vi "Misura res.vi"(6 "Scala per ramo":i32[](array[numeric]), 8 "String":string="Misura resistenze.. ", 9 "Status":refnum<vi>, 11 "N°rami":i32=3) -> (1 "temperature amb":dbl[](array[numeric]), 2 "Valori res (ohm)":dbl[](array[numeric]), 3 "Rmedia (ohm)":dbl format="%0.2f")   [LabVIEW 2019]
uses:
  cDAQ_PLC Folder/cDAQ/SET ARRAY DO.ctl
  cDAQ_PLC Folder/cDAQ/SET SINGLE DO.ctl
  cDAQ_PLC Folder/cDAQ/DO List.ctl
  <vilib>/Analysis/baseanly.llb/Mean (DBL).vi
  Global_All_Data.vi
  Global_scelta_linea.vi
  Resistomat/Stop lettura res.vi
  Global prova in corso.vi
  <vilib>/Analysis/NI_AALBase.lvlib
panel:
  in  "Scala di misura":u16
  out "Message":string
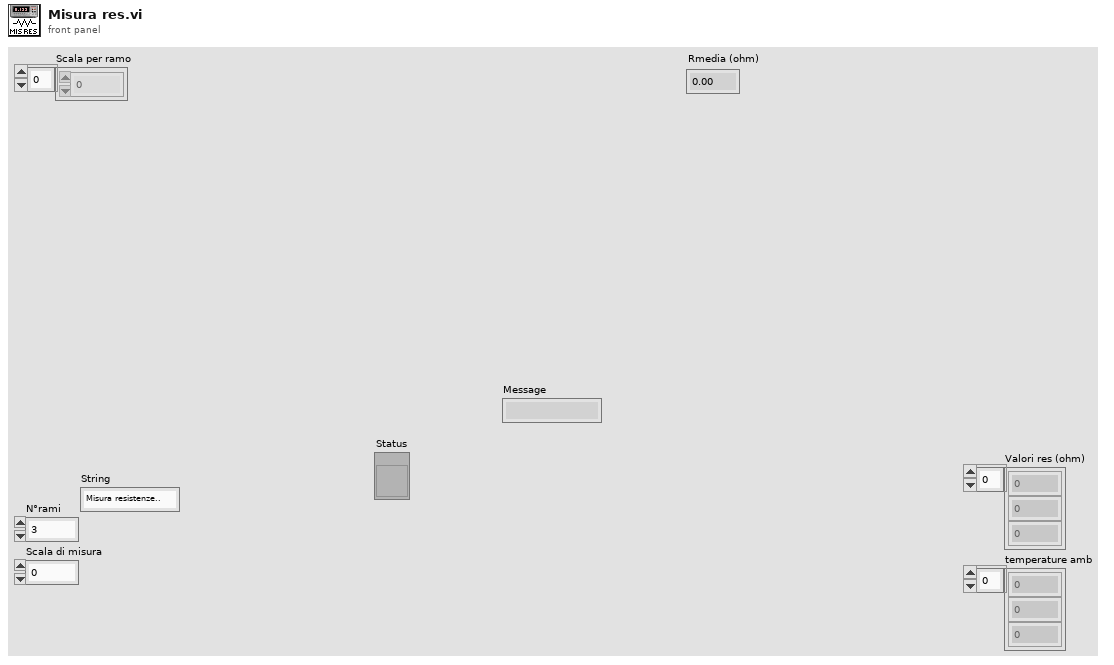
[diagram p1: front panel]
types:
  T1 = typedef "SET ARRAY DO.ctl" = T2[]
  T2 = typedef "SET SINGLE DO.ctl" = cluster{"DO":T3, "Value":bool}
  T3 = typedef "DO List.ctl" = enum16{"OFF: ALL DO", "*ABILITA freno 1", "*ABILITA freno 2", "*ABILITA freno 3", "*START freno 1", "*START freno 2", "*START freno 3", "*STOP freno 1", "*STOP freno 3", "*STOP freno 2", "*Senso rot freno 1", "*Senso rot freno 2", "*Senso rot freno 3", "*Ctrl velocità freno 1", "*Ctrl velocità freno 2", "*Ctrl velocità freno 3", "*Ctrl coppia freno 1", "*Ctrl coppia freno 2", "*Ctrl coppia freno 3", "*ABILITA alimentatore 1", "*ABILITA alimentatore 2", "*ABILITA alimentatore 3", "*ABILITA alimentatore 4", "*START alimentatore 1", "*START alimentatore 2", "*START alimentatore 3", "*START alimentatore 4", "*STOP alimentatore 1", "*STOP alimentatore 2", "*STOP alimentatore 3", "*STOP alimentatore 4", "SENSO ROT alimentatore 1", "SENSO ROT alimentatore 2", "Abilita LEM 1000A", "Abilita LEM 300A", "Abilita sensori EXT WT", "B1 Seleziona linea 1", "B1 Seleziona linea 2", "B1 Seleziona linea 3", "B1 Seleziona linea 4", "B1 Seleziona linea 5", "B2 Seleziona linea 1", "B2 Seleziona linea 2", "B2 Seleziona linea 3", "B2 Seleziona linea 4", "B2 Seleziona linea 5", "*Reset allarmi", "*Start potenza AC", "*Stop potenza AC", "*Start potenza DC", "*Stop potenza DC", "*Start potenza DC eccit", "*Stop pontenza DC eccit", "Bypass res meter", "2nd canale res meter", "Enable res meter", "*Abilit teler ramo WT", "*Abil teler ramo princ Resit", "*Abil teler ramo 1 Resist", "*Abil teler ramo 2 Resist", "*Abil teler ramo 3 Resist", "*Abil cortocirc avvolgim", "*Controllo torsiometro B1", "*Controllo Torsiom B2", "*Scala torsiometro B1", "*Scala torsiometro B2", "*Collaudo in corso", "*Allarme presente", "Abilitazione elettroserratura", "Exit", "*Abilita collaudo", "*Abilita potenza trifase", "*Abilita potenza monofase", "*Abilita potenza DC", "*Abilita potenza DC eccit", "*Disabilita teleruttori potenza", "Set teleruttori prova a freddo", "Prova a freddo monofase", "Watchdog", "Forza DO PLC 3", "Forza DO PLC 2", "Forza DO PLC 1", "Forza DO cDAQ", "Scala 2000(T) 200(F) res meter", "Seleziona banco 1", "Seleziona banco 2", "Comando azionam in blocco", "Comando azionam reset", "Sensibilità freno 16 32 nm", "Reset Allarmi", "Carico res - Ramo 1", "Carico res - Ramo 2", "Carico res - Ramo 3", "Carico res - Ramo 4", "Carico res - Ramo 5", "Carico res - Ramo 6", "Carico res - Ramo 7", "Carico res - Ramo 8", "Carico res - Ramo 9", "Carico res - Ramo 10", "Carico res - Ramo 11", "Carico res - Start ventilatore", "Carico res - Stop ventilatore", "Abilita potenza solo freno", "Abilita AFE + freno trasc", "Abilita potenza carico resistivo", "Chiudi potenza AFE", "Apri potenza AFE", "Start AFE", "Config Banco2 TDE", "Misura diretto WT", "Ripristina centralina protezioni", "Abilita Scrittura Dati Keb"}
  T4 = cluster{"Array of elements":cluster{"String":string, "variant":variant}[], "Single element":cluster{"String":string, "variant":variant}, "enque at\nopposite end (F)":bool, "no replications (F)":bool}
  T5 = typedef "Cluster MISURE.ctl" = cluster{"MISURE NM":T6, "MISURE ALL":T7}
  T6 = typedef "MISURE NM.ctl" = cluster{"Banco":string, "Anno":string, "Numero":string, "Ntabella":string, "Misura":string, "Tipo Prova":string, "ProgressivoAcq":string, "Descrizione":string, "Data_ora":string, "t. acq [h:m:s]":string, "t. acq [min]":string, "t. acq [s]":string, "n [rpm]":string, "f [Hz]":string, "U1[V]":string, "U2 [V]":string, "U3 [V]":string, "U123_media [V]":string, "I1[A]":string, "I2[A]":string, "I3[A]":string, "I123_media [A]*I":string, "I_123_sbil [%]":string, "Ulin[V]":string, "Uc [V]":string, "Uaux [V]":string, "Ilin[A]*I":string, "Imar[A]":string, "Iaux[A]":string, "Uarm[V]":string, "Uecc[V]":string, "Iarm[A]*I":string, "Iecc[A]":string, "pf":string, "P1 [W]":string, "P1 [kW]":string, "Q [VAR]":string, "Q [kVAR]":string, "S [VA]":string, "S [kVA]":string, "P1arm[W]":string, "P1ecc[W]":string, "Parm[kW]":string, "P1ecc[kW]":string, "Cond[uF]":string, "P1_linea_6fili[W]":string, "P1_linea_6fili[kW]":string, "eta_gr_6fili [%]":string, "eta_inverter_6fili [%]":string, "pf_linea_6fili":string, "U4 [V]":string, "U5 [V]":string, "U6 [V]":string, "U456_media [V]":string, "I4 [A]":string, "I5 [A]":string, "I6 [A]":string, "I456_media [A]":string, "C [Nm]*C":string, "Cric [Nm]":string, "Cric\\Cnom":string, "Iric[A]":string, "Iric\\Inom":string, "P2_mecc [W]":string, "P2_mecc [kW]":string, "eta motore [%]":string, "Scorr[%]":string, "Tamb[°C]":string, "R1[ohm]":string, "R2[ohm]":string, "R3[ohm]":string, "Rmedia[ohm]":string, "DT_R1[°C]":string, "DT_R2[°C]":string, "DT_R3[°C]":string, "DT_media[°C]":string, "R_marcia[ohm]":string, "R_aux[ohm]":string, "DT_marcia[°C]":string, "DT_aux[°C]":string, "R_Arm[ohm]":string, "R_Ecc[ohm]":string, "DT_Arm[°C]":string, "DT_Ecc[°C]":string, "TambFreddo[°C]":string, "R1_freddo[ohm]":string, "R2_freddo[ohm]":string, "R3_freddo[ohm]":string, "Rmedia_freddo[ohm]":string, "R_Marcia_freddo[ohm]":string, "R_Aux_freddo[ohm]":string, "R_Arm_freddo[ohm]":string, "R_Ecc_freddo[ohm]":string, "TC1 [°C]":string, "TC2 [°C]":string, "TC3 [°C]":string, "TC4 [°C]":string, "TC5 [°C]":string, "TC6 [°C]":string, "TC7 [°C]":string, "TC8 [°C]":string, "PT1000_1[°C]":string, "PT1000_2[°C]":string, "PT1000_3[°C]":string, "Vdc eccitatrice[V]":string, "Idc eccitatrice[A]":string, "Vdc rotore[V]":string, "Idc rotore[A]":string, "Vac rotore[V]":string, "Iac rotore[V]":string, "V dinamo[V]":string, "Portata Q":string, "Pressione H":string, "U1'[V]":string, "U2'[V]":string, "U3'[V]":string, "I1'[A]":string, "I2'[A]":string, "I3'[A]":string, "U''R-N":string, "U''S-N":string, "U'' T-N":string, "U''R-S":string, "U''R-T":string, "U''S-T":string, "I1''[A]":string, "I2''[A]":string, "I3''[A]":string, "F''[Hz]":string, "P''[kW]":string, "CosFi''":string, "PT1000_4[°C]":string, "Scorta 3":string}
  T7 = typedef "Cluster misure ALL.ctl" = cluster{"Cluster READ NI":T8, "MISURE WT":T11, "Resistenze Resistomat":T12, "INTERFACCIA":T13, "FREDDO resistomat":cluster{"Res Ch1":dbl, "Res Ch2":dbl, "tAMB":dbl, "Res Ch3":dbl}, "STATO PLC 1":T18, "Res Ch2":dbl, "Res Ch2 2":dbl, "FREDDO res meter":cluster{"Res Ch1":dbl, "Res Ch2":dbl, "tAMB":dbl, "Res Ch3":dbl}, "Resistenze Res Meter":T12, "READ SINUS PENTA":T22, "STATO PLC 2":T23, "STATO PLC 3":T27, "DCREG":T31}
  T8 = typedef "Cluster NI.ctl" = cluster{"AI (0-10V)":cluster{"AI 0":dbl, "AI 1":dbl, "AI 2":dbl, "AI 3":dbl, "AI 4":dbl, "AI 5":dbl, "AI 6":dbl, "AI 7":dbl, "AI 8":dbl, "AI 9":dbl, "AI 10":dbl, "AI 11":dbl, "AI 12":dbl, "AI 13":dbl, "AI 14":dbl, "AI 15":dbl, "AI 16":dbl, "AI 17":dbl, "AI 18":dbl, "AI 19":dbl, "AI 20":dbl, "AI 21":dbl, "AI 22":dbl, "AI 23":dbl, "AI 24":dbl, "AI 25":dbl, "AI 26":dbl, "AI 27":dbl, "AI 28":dbl, "AI 29":dbl, "AI 30":dbl, "AI 31":dbl}, "StatoAO_Cdaq[0-10V]":cluster{"AO 1":dbl, "AO 2":dbl, "AO 3":dbl, "AO 4":dbl}, "Contatori [rpm]":cluster{"RPM 1":dbl, "RPM 2":dbl}, "StatoAO_Cdaq [4-20mA]":T9, "StatoDO_Cdaq":T10, "DI":cluster{"Scorta 0":bool, "Scorta 1":bool, "Scorta 2":bool, "Scorta 3":bool, "Scorta 4":bool, "Scorta 5":bool, "Scorta 6":bool, "Scorta 7":bool, "Scorta 8":bool, "Scorta 9":bool, "Scorta 10":bool, "Scorta 11":bool, "Scorta 12":bool, "Scorta 13":bool, "Scorta 14":bool, "Scorta 15":bool, "Scorta 16":bool, "Scorta 17":bool, "Scorta 18":bool, "Scorta 19":bool, "Scorta 20":bool, "Scorta 21":bool, "Scorta 22":bool, "Scorta 23":bool, "Scorta 24":bool, "Scorta 25":bool, "Scorta 26":bool, "Scorta 27":bool, "Scorta 28":bool, "Scorta 29":bool, "Scorta 30":bool, "Scorta 31":bool}, "AI (4-20mA)":cluster{"AI 0":dbl, "AI 1":dbl, "AI 2":dbl, "AI 3":dbl, "AI 4":dbl, "AI 5":dbl, "AI 6":dbl, "AI 7":dbl, "AI 8":dbl, "AI 9":dbl, "AI 10":dbl, "AI 11":dbl, "AI 12":dbl, "AI 13":dbl, "AI 14":dbl, "AI 15":dbl}, "TC [°C]":cluster{"tc 1":dbl, "tc 2":dbl, "tc 3":dbl, "tc 4":dbl}}
  T9 = typedef "StatoAO_cdaq.ctl" = cluster{"Cdaq_AO [0-10V] 0":dbl, "Cdaq_AO [0-10V] 1":dbl, "Cdaq_AO [0-10V] 2":dbl, "Cdaq_AO [0-10V] 3":dbl, "Cdaq_AO [4-20mA] 0":dbl, "Cdaq_AO [4-20mA] 1":dbl, "Cdaq_AO [4-20mA] 2":dbl, "Cdaq_AO [4-20mA] 3":dbl, "Cdaq_AO [4-20mA] 4":dbl, "Cdaq_AO [4-20mA] 5":dbl, "Cdaq_AO [4-20mA] 6":dbl, "Cdaq_AO [4-20mA] 7":dbl}
  T10 = typedef "statoDO_Cdaq.ctl" = cluster{"Scorta 0":bool, "Scorta 1":bool, "Scorta 2":bool, "Scorta 3":bool, "Scorta 4":bool, "Scorta 5":bool, "Scorta 6":bool, "Scorta 7":bool, "Scorta 8":bool, "Scorta 9":bool, "Scorta 10":bool, "Scorta 11":bool, "Scorta 12":bool, "Scorta 13":bool, "Scorta 14":bool, "Scorta 15":bool, "Scorta 16":bool, "Scorta 17":bool, "Scorta 18":bool, "Scorta 19":bool, "Scorta 20":bool, "Scorta 21":bool, "Scorta 22":bool, "Scorta 23":bool, "Scorta 24":bool, "Scorta 25":bool, "Scorta 26":bool, "Scorta 27":bool, "Scorta 28":bool, "Scorta 29":bool, "Scorta 30":bool, "Scorta 31":bool}
  T11 = typedef "MISURE WT.ctl" = cluster{"URMS 1":dbl, "IRMS 1":dbl, "P 1":dbl, "S 1":dbl, "Q 1":dbl, "LAMBDA 1":dbl, "PHI 1":dbl, "F U 1":dbl, "F I 1":dbl, "NONE 1":dbl, "URMS 2":dbl, "IRMS 2":dbl, "P 2":dbl, "S 2":dbl, "Q 2":dbl, "LAMBDA 2":dbl, "PHI 2":dbl, "F U 2":dbl, "F I 2":dbl, "NONE 2":dbl, "URMS 3":dbl, "IRMS 3":dbl, "P 3":dbl, "S 3":dbl, "Q 3":dbl, "LAMBDA 3":dbl, "PHI 3":dbl, "F U 3":dbl, "F I 3":dbl, "NONE 3":dbl, "URMS 4":dbl, "IRMS 4":dbl, "P 4":dbl, "S 4":dbl, "Q 4":dbl, "LAMBDA 4":dbl, "PHI 4":dbl, "F U 4":dbl, "F I 4":dbl, "NONE 4":dbl, "URMS 5":dbl, "IRMS 5":dbl, "P 5":dbl, "S 5":dbl, "Q 5":dbl, "LAMBDA 5":dbl, "PHI 5":dbl, "F U 5":dbl, "F I 5":dbl, "NONE 5":dbl, "URMS 6":dbl, "IRMS 6":dbl, "P 6":dbl, "S 6":dbl, "Q 6":dbl, "LAMBDA 6":dbl, "PHI 6":dbl, "F U 6":dbl, "F I 6":dbl, "NONE 6":dbl, "URMS SIGMA":dbl, "IRMS SIGMA":dbl, "P SIGMA":dbl, "S SIGMA":dbl, "Q SIGMA":dbl, "LAMBDA SIGMA":dbl, "PHI SIGMA":dbl, "F U SIGMA":dbl, "F I SIGMA":dbl, "NONE 7":dbl, "URMS SIGMB":dbl, "IRMS SIGMB":dbl, "P SIGMB":dbl, "S SIGMB":dbl, "Q SIGMB":dbl, "LAMBDA SIGMB":dbl, "PHI SIGMB":dbl, "F U SIGMB":dbl, "F I SIGMB":dbl, "NONE 8":dbl, "URMS SIGMC":dbl, "IRMS SIGMC":dbl, "P SIGMC":dbl, "S SIGMC":dbl, "Q SIGMC":dbl, "LAMBDA SIGMC":dbl, "PHI SIGMC":dbl, "F U SIGMC":dbl, "F I SIGMC":dbl, "NONE 9":dbl, "SPEED":dbl, "TORQUE[Nm]":dbl, "Pmecc[kW]":dbl}
  T12 = typedef "ClusterRes.ctl" = cluster{"Res Ch1":dbl, "Res Ch2":dbl, "Res Ch3":dbl, "Tamb":dbl}
  T13 = typedef "INTERFACCIA.ctl" = cluster{"AI":cluster{"Portate":T14[], "Pressioni":T14[], "Coppie[Nm]":T14[], "Valvole prop %":T14[], "RPM":T14[], "Livelli":T14[], "Temperature":T14[], "Riferimenti %":T14[], "TENSIONI":T14[], "CORRENTI":T14[]}, "DI (logici)":cluster{"Start da pulsantiera":bool, "Stop da pulsantiera":bool, "Reset da pulsantiera":bool, "Sistema OK":bool, "Collaudo abilitato":bool, "Potenza trifase abilitata":bool, "Potenza monofase abilitata":bool, "Potenza DC abilitata":bool, "Potenza DC ECC abilitata":bool, "Start alimentazione AC":bool, "Start alimentazione DC":bool, "Start DC eccitazione":bool, "Teleruttore WT abilitato":bool, "Teleruttore Resistomat abilitato":bool, "Teleruttore corto fasi":bool, "Ramo 1 resistomat":bool, "Ramo 2 resistomat":bool, "Ramo 3 resistomat":bool, "B1 Scelta linea elettrica 1":bool, "B1 Scelta linea elettrica 2":bool, "B1 Scelta linea elettrica 3":bool, "B1 Scelta linea elettrica 4":bool, "B1 Scelta linea elettrica 5":bool, "B2 Scelta linea elettrica 1":bool, "B2 Scelta linea elettrica 2":bool, "B2 Scelta linea elettrica 3":bool, "B2 Scelta linea elettrica 4":bool, "B2 Scelta linea elettrica 5":bool, "Rotore bloccato 1":bool, "Rotore bloccato 2":bool, "FRENO 1 abilitato":bool, "FRENO 1 run":bool, "FRENO 1 senso rotaz":bool, "FRENO 1 ctrl velocità":bool, "FRENO 2 abilitato":bool, "FRENO 2 run":bool, "FRENO 2 senso rotaz":bool, "FRENO 2 ctrl velocità":bool, "ALIM 1 abilitato":bool, "ALIM 1 run":bool, "ALIM 2 abilitato":bool, "ALIM 2 run":bool, "ALIM 3 abilitato":bool, "ALIM 3 run":bool, "FRENO 1 ctrl coppia":bool, "FRENO 2 ctrl coppia":bool, "FRENO 3 ctrl coppia":bool, "DI (logici) aggiuntivi impianto":cluster{"Solo freno abilitato":bool, "Carico resistivo abilitato":bool, "AFE+freno abilitato":bool, "Protezioni chiuse":bool, "Start potenza AFE":bool, "AFE in marcia":bool}, "Misura corrente diretta WT":bool, "Misura corrente sens ext":bool, "Sens ext abilitati":bool}, "AO non scalati":T16, "AO scalati":T16, "DO (logici)":T17}
  T14 = typedef "ClusterMisura_e_Unità_INPUT.ctl" = cluster{"Misura":dbl, "UM":T15, "Descrizione":string}
  T15 = typedef "UnitàMisura.ctl" = enum16{"V", "mA", "Bar", "RPM", "m3/s", "m3/min", "m3/h", "l/s", "l/min", "in3/min", "ft3/min", "gpm", "igpm", "igph", "%", "°C", "m", "Nm", "A"}
  T16 = typedef "Lista AO sistema.ctl" = cluster{"FRENO1 rif vel":dbl, "FRENO1 rif Coppia":dbl, "FRENO2 rif vel":dbl, "FRENO2 rif Coppia":dbl, "ALIM1 rif V":dbl, "ALIM1 rif F":dbl, "ALIM2 rif V":dbl, "ALIM2 rif F":dbl, "ALIM3 rif V":dbl, "ALIM3 rif F":dbl, "Fnom keb":dbl, "Rpm nom keb":dbl, "Pnom keb":dbl, "Inom keb":dbl, "Vnom keb":dbl, "Rpm max keb":dbl, "Tempo rampa keb":dbl, "Tipo Mot keb":dbl}
  T17 = typedef "DOinterfaccia.ctl" = cluster{"Scelta banco 1":bool, "Scelta banco 2":bool, "Scelta banco 3":bool, "FRENO 1 abilita":bool, "FRENO 1 start":bool, "FRENO 1 senso rotaz":bool, "FRENO 1 ctrl velocità":bool, "FRENO 2 abilita":bool, "FRENO 2 start":bool, "FRENO 2 senso rotaz":bool, "FRENO 2 ctrl velocità":bool, "ALIM 1 abilita":bool, "ALIM 1 start":bool, "ALIM 2 abilita":bool, "ALIM 2 start":bool, "ALIM 3 abilita":bool, "ALIM 3 start":bool, "Abilita linea trifase":bool, "Abilita linea monofase":bool, "Abilita linea dc":bool, "Abilita linea dc eccit":bool, "B1 Linea elettrica 1":bool, "B1 Linea elettrica 2":bool, "B1 Linea elettrica 3":bool, "B1 Linea elettrica 4":bool, "B1 Linea elettrica 5":bool, "B2 Linea elettrica 1":bool, "B2 Linea elettrica 2":bool, "B2 Linea elettrica 3":bool, "B2 Linea elettrica 4":bool, "B2 Linea elettrica 5":bool, "Start potenza AC":bool, "Stop pontenza AC":bool, "Start potenza DC":bool, "Stop potenza DC":bool, "Start potenza eccitaz":bool, "Stop potenza eccitaz":bool, "Reset allarmi":bool, "watchdog":bool, "Scala torsiometro B1":bool, "Controllo torsiom B1":bool, "Scala torsiometro B2":bool, "Controllo torsiom B2":bool, "Teleruttore WT abilita":bool, "Teleruttore Resistomat abilita":bool, "Teleruttore corto fasi":bool, "Ramo 1 resistomat":bool, "Ramo 2 resistomat":bool, "Ramo 3 resistomat":bool, "Collaudo in corso":bool, "Allarme presente":bool, "Enable Res Meter":bool, "Bypass Res Meter":bool, "2nd canale Res Meter":bool, "Scala 200/2000 res meter":bool, "Taratura res meter":bool, "FRENO 1 ctrl coppia":bool, "FRENO 2 ctrl coppia":bool, "FRENO 3 ctrl coppia":bool, "Aggiuntivi impianto":cluster{"Senso rotazione alim 1":bool, "Senso rotazione alim 2":bool}, "ALIM 1 stop":bool, "ALIM 2 stop":bool, "ALIM 3 stop":bool, "FRENO 1 stop":bool, "FRENO 2 stop":bool, "FRENO 3 stop":bool, "B1 configurazione freno B":bool, "B2 configurazione freno B":bool, "Abilita scrittura KEB":bool}
  T18 = typedef "STATO PLC 1.ctl" = cluster{"USCITE PLC":T19, "Stato DI_PLC":cluster{"Sistema OK":bool, "Rotore bloccato":bool, "Scorta 1":bool, "Prova diretto inverter":bool, "Prova con filtro LC":bool, "Teleruttore WT abilitato":bool, "Alim sinus penta abilitato":bool, "Alim sinus penta in marcia":bool, "Freno abilitato":bool, "Freno in marcia":bool, "Senso rotazione freno":bool, "Potenza abilitata":bool, "Scorta 3":bool, "Scorta 4":bool, "scorta 5":bool, "scorta 6":bool}, "AI plc":cluster{"Allarmi 1":dbl, "Allarmi 2":dbl, "Scorta 1":dbl, "Scorta 2":dbl, "RPM mot prova":dbl, "I mot prova":dbl, "RPM freno":dbl, "I freno":dbl, "Scorta 3":dbl, "Scorta 4":dbl}}
  T19 = typedef "Uscite PLC 1.ctl" = cluster{"AO (real) 2":cluster{"SCORTA 1":dbl, "SCORTA 2":dbl, "SCORTA 3":dbl, "SCORTA 4":dbl, "SCORTA 5":dbl, "SCORTA 6":dbl, "SCORTA 7":dbl, "SCORTA 8":dbl}, "statoAO_PLC out":T20, "DO (bit)":T21}
  T20 = typedef "statoAO_plc_1.ctl" = cluster{"Rif Lim coppia freno [%]":dbl, "Rif rpm freno [%]":dbl, "Rif coppia freno [%]":dbl, "Rif V alimentatore [%]":dbl, "Rif F alimentatore [%]":dbl}
  T21 = typedef "StatoDO_PLC_1.ctl" = cluster{"Scelta banco 1":bool, "Set dati motore freno 2":bool, "Diretto inverter":bool, "Filtro LC":bool, "Marcia ALIM (1s)":bool, "Marcia FRENO (1s)":bool, "Stop AFE (1s)":bool, "Stop freno (1s)":bool, "Reset allarmi":bool, "Watchdog":bool, "Senso rotazione":bool, "Abilita collaudo (1s)":bool, "Disabilita collaudo (1s)":bool, "Abilitazione ALIM":bool, "Abilitazione FRENO":bool, "Teleruttore WT":bool, "Senso rot motore prova":bool, "Scorta 7":bool, "Scorta 8":bool, "Scorta 9":bool, "Scorta 10":bool, "Scorta 11":bool, "Scorta 12":bool, "Scorta 13":bool}
  T22 = typedef "Parametri inverter letti.ctl" = cluster{"Menù Misure motore (M000-M030)":cluster{"Rif vel a regime (int)":u16, "Rif vel a regime (dec)":u16, "Rif vel dopo rampe (int)":u16, "Rif vel dopo rampe (dec)":u16, "RPM motore (int)":u16, "RPM motore (dec)":u16, "FREQout inverter":u16, "Rif coppia a regime(Nm)":u16, "Richiesta di coppia (Nm)":u16, "Coppia generata dal motore(Nm)":u16, "Rif coppia a regime(%)":u16, "Richiesta di coppia (%)":u16, "Coppia generata dal motore(%)":u16, "Coppia max richiesta prima delle rampe(Nm)":u16, "Coppia max richiesta dopo le rampe(Nm)":u16, "Limite di velocità prima delle rampe":u16, "Limite di velocità dopo le rampe":u16, "Coppia max richiesta prima delle rampe(%)":u16, "Coppia max richiesta dopo le rampe(%)":u16, "Rif di flusso":u16, "Corrente di uscita":u16, "Capacità termica del motore":u16, "Tensione di uscita":u16, "Potenza di uscita":u16, "Energia consumata (LSword)":u16, "Energia consumata (MSword)":u16, "Tensione bus DC":u16, "Tensione di rete":u16}, "Menù regolatore PID (M018-M024)":cluster{"Rif PID a regime(%)":u16, "Rif pid dopo rampe(%)":u16, "Retroazione del pid(%)":u16, "Errore del pid(%)":u16, "uscita del pid(%)":u16, "Rif del pid dopo le rampe":u16, "Retroazione del pid":u16}, "Menù ingressi digitali (M031-M036)":cluster{"Ingressi digitali ritardati":u16, "Ingressi digitali istantanei":u16, "Moresettiera comando loc":u16, "Morsett comando da seriale":u16, "Morsett comando bus di campo":u16, "Ing dig ausiliari da morsettiera":u16, "Ing dig ausiliari da seriale":u16}, "Menù riferimenti (M037-M051)":cluster{"Rif analog est REF":u16, "Rif analog est AIN1":u16, "Rif analog est AIN2":u16, "Rif analog est XAIN4":u16, "Rif analog est XAIN5":u16, "Rif velocità da seriale(int)":u16, "Rif velocità bus di campo(int)":u16, "Rif coppia da seriale":u16, "Rif coppia bus di campo":u16, "Rif del PID da seriale":u16, "Rif del PID da bus di campo":u16, "Retroazione del PID da seriale":u16, "Retroazione del PIDda bus di campo":u16, "Rif da encoder":u16, "Rif in frequenza":u16, "Rif velocità da seriale(dec)":u16, "Rif velocità bus di campo(dec)":u16}, "Menù rampe (P009-P033)":cluster{"Tempo di dec rampa di vel 1":u16, "Tempo di acc rampa di vel 2":u16, "Tempo di dec rampa di vel 2":u16, "Tempo di acc rampa di vel 1":u16, "Unità di mis tempi rampe vel 1/2":u16, "Tempo di acc rampa di vel 3":u16, "Tempo di dec rampa di vel 3":u16, "Tempo di acc rampa di vel 4":u16, "Tempo di dec rampa di vel 4":u16, "Unità di mis tempi rampe vel 3/4":u16, "Selettore arrottondam rampe":u16, "Tempo di arrotond iniz rampa acc":u16, "Tempo di arrotond finale rampa acc":u16, "Tempo di arrotond iniz rampa dec":u16, "Tempo di rampa di salita rif coppia":u16, "Tempo di rampa di discesa rif coppia":u16, "Unità di misura rampa coppia":u16, "Tempo rampa acc marcia jog":u16, "Tempo rampa dec marcia jog":u16, "Reset acc ai cambi pendenza":u16, "rampa di acc in fire mode":u16, "rampa di dec in fire mode":u16, "Tempo di arrotond finale rampa dec":u16}, "Menù controllo motore(C008-C128)":cluster{"Numero motori configurati":u16, "Tipo algoritmo di controllo Mot1":u16, "Tipo rif Mot1":u16, "Tensione nominale rete":u16, "Retroaz di vel da encoder Mot1":u16, "Tipo curva V/f Mot1":u16, "Rotazione delle fasi Mot1":u16, "Freq nominale del motore Mot1":u16, "RPM nominali del motore Mot1":u16, "Potenza nominale del motore Mot1":u16, "Corrente nominale del motore Mot1":u16, "Tensione nominale del motore mot1":u16, "Potenza a vuoto del motore Mot1":u16, "Corrente a vuoto del motore Mot1":u16, "Resistenza statorica del motore Mot1":u16, "Induttanza di dispersione Mot1":u16, "Induttanza mutua motore":u16, "Costante di tempo rotorica":u16, "Costante di tempo filtro pb":u16, "Velocità minima motore":u16, "Velocità massima motore":u16}, "Menù configurazione PID":cluster{"Selezione riferimento n.1":u16, "Selezione retroazione n.1":u16, "Modalità di fuzionamento PID":u16, "Termine derivativo calcolato su err o mis":u16, "Proporz moltiplica deriv e integrale":u16, "Azione del PID":u16}, "ID":dbl, "Menù uscite digitali":cluster{"MDO4 Inverter pronto":u16}, "Fcarrier":cluster{"Fcarrier Min (Hz)":u16, "Fcarrier Max (Hz)":u16}, "stato inverter M089":dbl, "Riferimenti":cluster{"Rif tensione":u16, "Rif velocità":u16}, "Comunicazione":bool, "Modalità stop":dbl}
  T23 = typedef "STATO PLC 2.ctl" = cluster{"USCITE PLC":T24, "Stato DI_PLC":cluster{"Sistema ok":bool, "Relè Resistomat abilitato":bool, "scorta d":bool, "scorta c":bool, "scorta b":bool, "scorta a":bool, "scorta 1":bool, "scorta 2":bool, "scorta 3":bool, "scorta 4":bool, "Scorta 5":bool, "Scorta 6":bool, "Scorta 7":bool, "Scorta 8":bool, "Scorta 9":bool, "Scorta 10":bool}, "AI plc":cluster{"Allarmi 1":dbl, "Allarmi 2":dbl, "TC 1":dbl, "TC 2":dbl, "TC 3":dbl, "TC 4":dbl, "TC 5":dbl, "TC 6":dbl, "TC 7":dbl, "TC 8":dbl, "PT1000 1":dbl, "PT1000 2":dbl, "PT1000 3":dbl, "PT1000 4":dbl}}
  T24 = typedef "Uscite PLC 2.ctl" = cluster{"AO (real) 2":cluster{"SCORTA 1":dbl, "SCORTA 2":dbl, "SCORTA 3":dbl, "SCORTA 4":dbl, "SCORTA 5":dbl, "SCORTA 6":dbl, "SCORTA 7":dbl, "SCORTA 8":dbl}, "statoAO_PLC out":T25, "DO (bit)":T26}
  T25 = typedef "statoAO_plc_2.ctl" = cluster{"Condensatori":dbl, "Scorta 1":dbl, "Scorta 2":dbl}
  T26 = typedef "StatoDO_PLC_2.ctl" = cluster{"Scala Torsiometro":bool, "Ctrl torsiometro":bool, "Relè misura resistomat":bool, "Watchdog":bool, "Misura res ramo 1":bool, "Misura res ramo 2":bool, "Misura res ramo 3":bool, "Scelta banco 2":bool, "Reset allarmi":bool, "Reset centraline":bool, "Scorta 2":bool, "Scorta 3":bool, "Scorta 4":bool, "Scorta 5":bool, "Scorta 6":bool, "Scorta 7":bool}
  T27 = typedef "STATO PLC 3.ctl" = cluster{"USCITE PLC":T28, "Stato DI_PLC":cluster{"Sistema OK":bool, "Rotore bloccato":bool, "Filtro LC":bool, "Bypass Filtro LC":bool, "Scelta Trasformatore":bool, "Scelta Bypass trasformatore":bool, "Teleruttore wt abilitato":bool, "Alimentatore abilitato":bool, "Alimentatore in marcia":bool, "Freno abilitato":bool, "Freno in marcia":bool, "Freno senso di rotazione":bool, "Potenza abilitata":bool, "Alimentatore in allarme":bool, "Freno in allarme":bool, "Conferma dati KEB":bool, "Scorta 4":bool, "Scorta 5":bool, "Scorta 6":bool}, "AI plc":cluster{"Allarmi 1":dbl, "Allarmi 2":dbl, "RPM motore prova":dbl, "Corrente motore prova":dbl, "RPM freno":dbl, "Corrente freno":dbl, "Tipo motore keb":dbl, "I nom keb":dbl, "RPM nom keb":dbl, "V nom keb":dbl, "F nom keb":dbl, "T rampa keb":dbl, "scorta":dbl, "Scorta 2":dbl}}
  T28 = typedef "Uscite PLC 3.ctl" = cluster{"AO (real) 2":cluster{"SCORTA 1":dbl, "SCORTA 2":dbl, "SCORTA 3":dbl, "SCORTA 4":dbl, "SCORTA 5":dbl, "SCORTA 6":dbl, "SCORTA 7":dbl, "SCORTA 8":dbl}, "statoAO_PLC out":T29, "DO (bit)":T30}
  T29 = typedef "statoAO_plc_3.ctl" = cluster{"Rif limitazione coppia freno":dbl, "Rif velocità freno":dbl, "Rif coppia freno (predisp.)":dbl, "Rif velocità alimentatore":dbl, "Scorta":dbl, "Tipo Motore  keb":dbl, "I nom keb":dbl, "RPM nom keb":dbl, "V nom keb":dbl, "F nom keb":dbl, "t rampa keb":dbl, "scorta":dbl, "Scorta 2":dbl}
  T30 = typedef "StatoDO_PLC_3.ctl" = cluster{"Scelta banco 2":bool, "Abilita Scrittura Dati Keb":bool, "Filtro LC":bool, "Bypass filtro LC":bool, "Trasformatore":bool, "Bypass trasformatore":bool, "Marcia alimentatore (1s)":bool, "Marcia freno (1s)":bool, "Stop alimentatore (1s)":bool, "Stop freno (1s)":bool, "Reset allarmi":bool, "Watchdog":bool, "Freno senso di rotazione":bool, "Abilita pontenza (1s)":bool, "Disabilita potenza (1s)":bool, "Abilita alimentatore":bool, "Abilita freno":bool, "Teleruttore wt":bool, "Senso rot mot prova":bool, "Scorta":bool, "Scorta":bool, "Blocco elettroserrature":bool, "Scorta 6":bool, "Scorta 7":bool}
  T31 = typedef "Parametri DCREG letti.ctl" = cluster{"Parametri di misura":cluster{"M000":dbl, "M001":dbl, "M002":dbl, "M003":dbl, "M004":dbl, "M005":dbl, "M006":dbl, "M007":dbl, "M008":dbl, "M009":dbl, "M010":dbl, "M011":dbl, "M012":dbl, "M013":dbl, "M014":dbl, "M015":dbl, "M016":dbl, "M017":dbl, "M018":dbl, "M019":dbl, "M020":dbl, "M021":dbl, "M022":dbl, "M023":dbl, "M024":dbl, "M025":dbl, "M026":dbl, "M027":dbl, "M028":dbl, "M029":dbl, "M030":dbl, "M031":dbl}, "Parametri di programmazione":cluster{"P000":dbl, "P001":dbl, "P002":dbl, "P003":dbl, "P004":dbl, "P005":dbl, "P006":dbl, "P010":dbl, "P011":dbl, "P012":dbl, "P013":dbl, "P014":dbl, "P015":dbl, "P016":dbl, "P030":dbl, "P031":dbl, "P032":dbl, "P033":dbl, "P034":dbl, "P035":dbl, "P036":dbl, "P037":dbl, "P038":dbl, "P039":dbl, "P040":dbl, "P050":dbl, "P051":dbl, "P052":dbl, "P053":dbl, "P054":dbl, "P055":dbl, "P056":dbl, "P057":dbl, "P058":dbl, "P059":dbl, "P060":dbl, "P061":dbl, "P062":dbl, "P070":dbl, "P071":dbl, "P073":dbl, "P074":dbl, "P076":dbl, "P077":dbl, "P079":dbl, "P080":dbl, "P082":dbl, "P083":dbl, "P084":dbl, "P085":dbl, "P086":dbl, "P087":dbl, "P088":dbl, "P100":dbl, "P101":dbl, "P102":dbl, "P103":dbl, "P104":dbl, "P110":dbl, "P111":dbl, "P120":dbl, "P121":dbl, "P122":dbl, "P123":dbl, "P124":dbl, "P125":dbl, "P126":dbl, "P127":dbl, "P128":dbl, "P129":dbl, "P130":dbl, "P131":dbl, "P132":dbl, "P133":dbl, "P134":dbl, "P150":dbl, "P151":dbl, "P152":dbl, "P153":dbl, "P154":dbl, "P155":dbl, "P156":dbl, "P157":dbl, "P158":dbl, "P170":dbl, "P171":dbl, "P172":dbl, "P173":dbl, "P174":dbl, "P175":dbl, "P176":dbl, "P177":dbl, "P178":dbl, "P179":dbl, "P180":dbl, "P181":dbl, "P182":dbl, "P183":dbl, "P184":dbl, "P185":dbl, "P186":dbl, "P187":dbl, "P188":dbl, "P189":dbl, "P190":dbl, "P191":dbl, "P192":dbl, "P193":dbl, "P194":dbl, "P195":dbl, "P196":dbl, "P197":dbl, "P198":dbl, "P199":dbl, "P211":dbl, "P212":dbl, "P213":dbl, "P214":dbl, "P215":dbl, "P216":dbl, "P217":dbl, "P221":dbl, "P222":dbl, "P223":dbl, "P224":dbl, "P230":dbl, "P231":dbl, "P240":dbl, "P250":dbl, "P251":dbl}, "Parametri di configurazione":cluster{"C000":dbl, "C001":dbl, "C002":dbl, "C010":dbl, "C011":dbl, "C012":dbl, "C014":dbl, "C015":dbl, "C016":dbl, "C017":dbl, "C018":dbl, "C030":dbl, "C050":dbl, "C051":dbl, "C052":dbl, "C060":dbl, "C061":dbl, "C062":dbl, "C063":dbl, "C070":dbl, "C072":dbl, "C074":dbl, "C090":dbl, "C091":dbl, "C092":dbl, "C093":dbl, "C094":dbl, "C100":dbl, "C101":dbl, "C102":dbl, "C103":dbl, "C105":dbl, "C106":dbl, "C107":dbl, "C108":dbl, "C110":dbl, "C111":dbl, "C112":dbl, "C120":dbl, "C121":dbl, "C122":dbl, "C130":dbl, "C131":dbl, "C132":dbl, "C133":dbl, "C134":dbl, "C135":dbl, "C141":dbl, "C142":dbl, "C143":dbl, "C150":dbl, "C151":dbl, "C153":dbl, "C154":dbl, "C155":dbl, "C156":dbl, "C157":dbl, "C158":dbl, "C159":dbl, "C160":dbl, "C161":dbl, "C162":dbl, "C163":dbl, "C164":dbl, "C165":dbl, "C170":dbl}, "Codice allarme":dbl, "Comunicazione":bool}
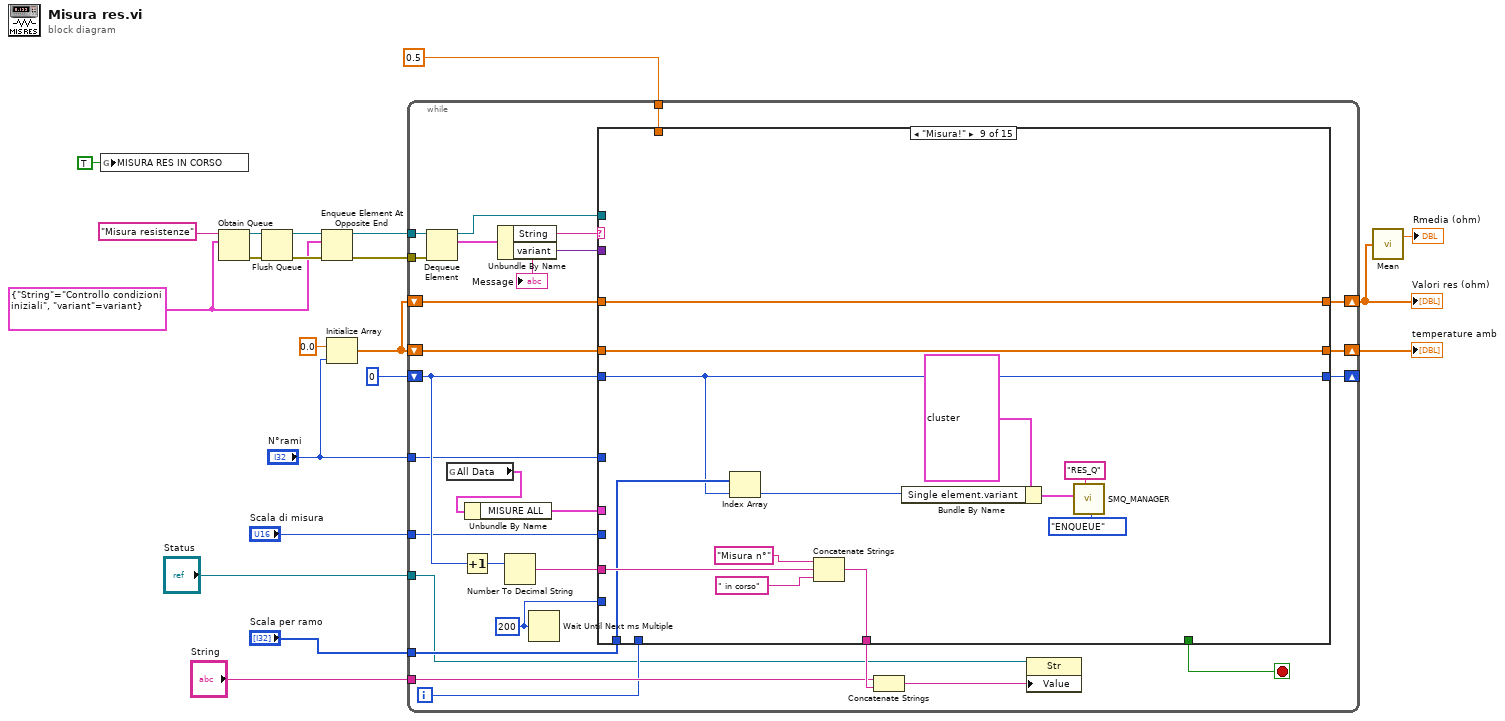
[diagram p0: block diagram]
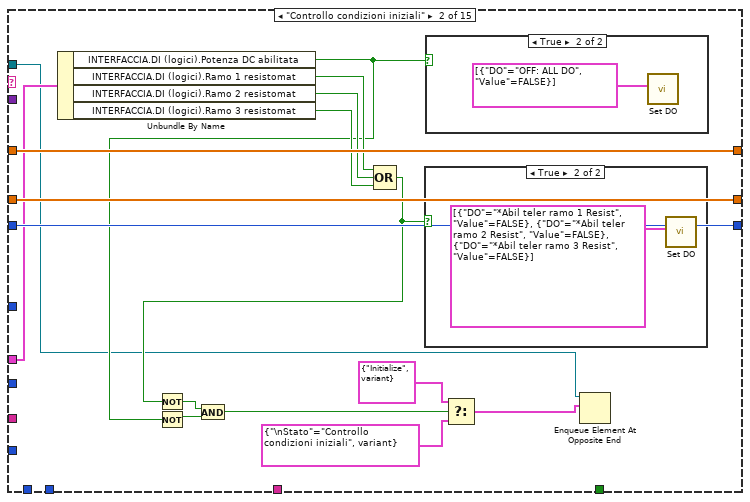
[diagram p3: hidden frame]
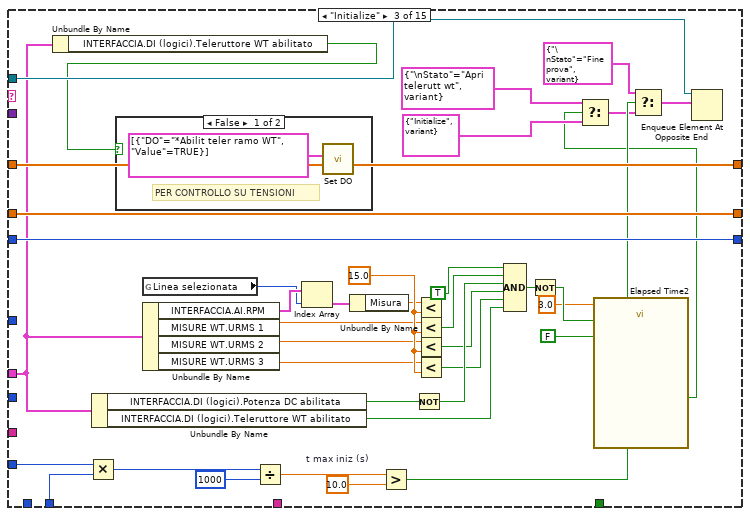
[diagram p6: hidden frame]
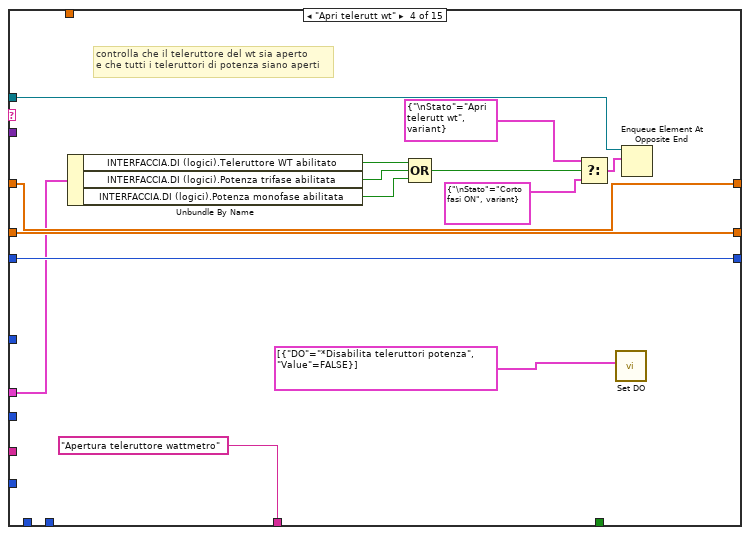
[diagram p8: hidden frame]
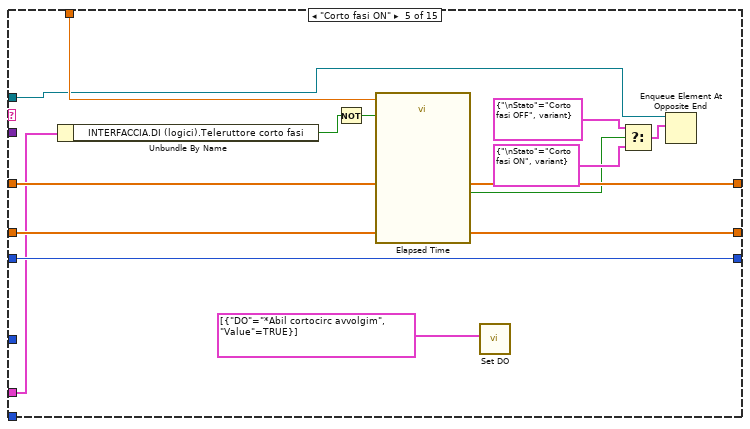
[diagram p9: hidden frame]
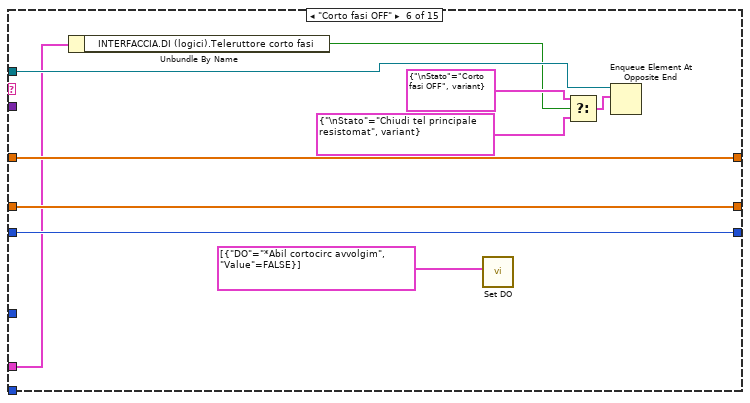
[diagram p10: hidden frame]
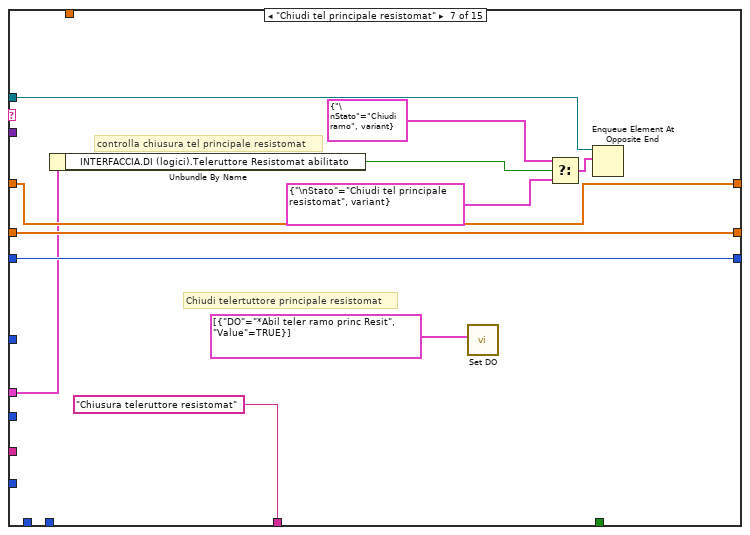
[diagram p11: hidden frame]
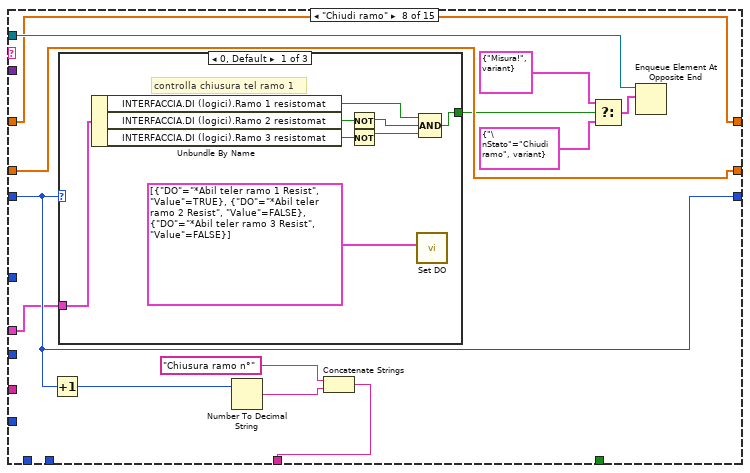
[diagram p12: hidden frame]
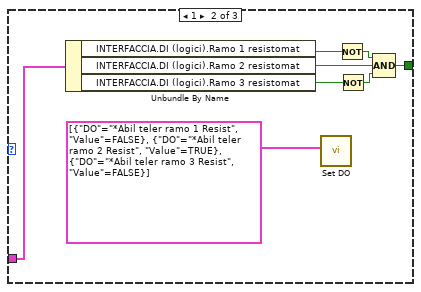
[diagram p13: hidden frame]
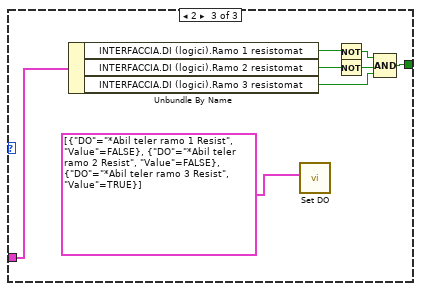
[diagram p14: hidden frame]
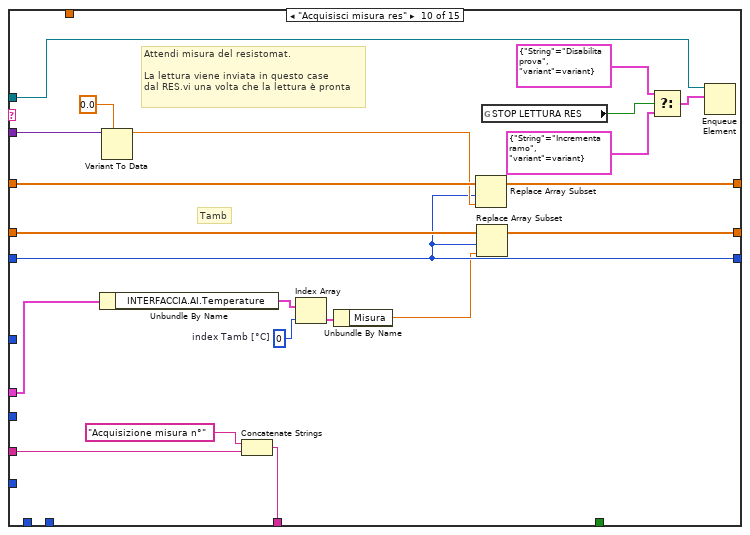
[diagram p15: hidden frame]
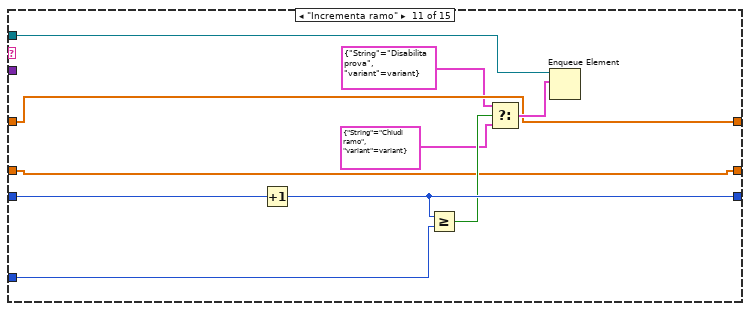
[diagram p16: hidden frame]
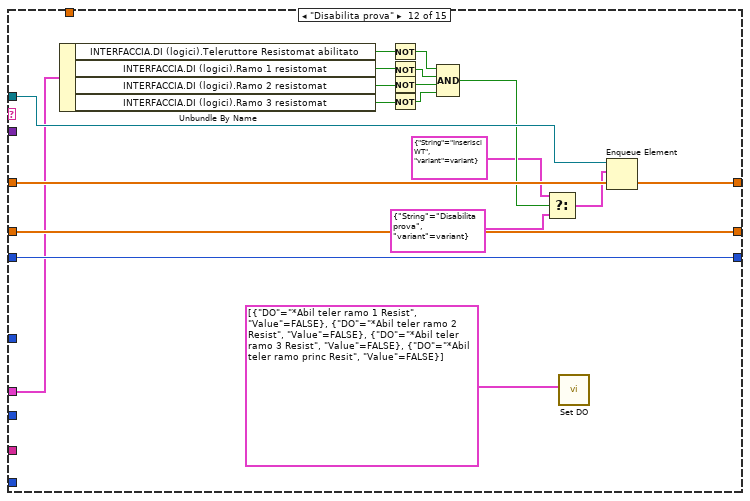
[diagram p17: hidden frame]
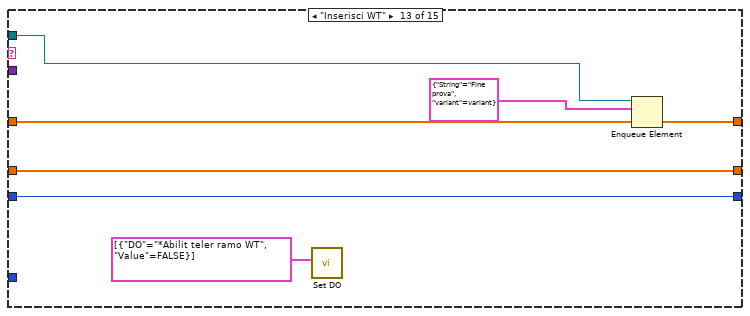
[diagram p18: hidden frame]
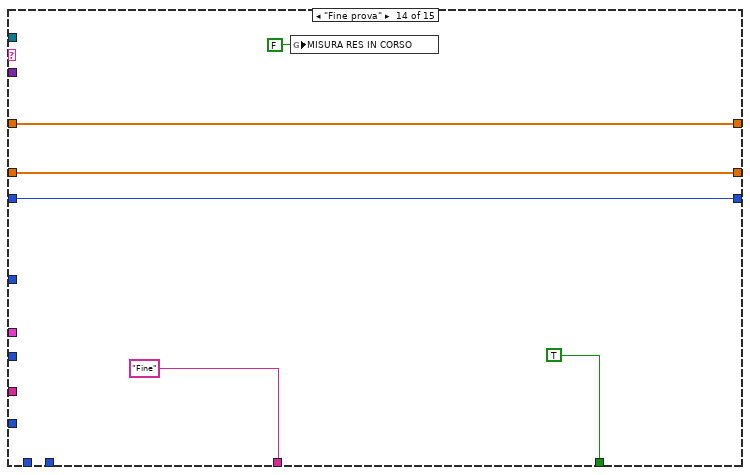
[diagram p19: hidden frame]
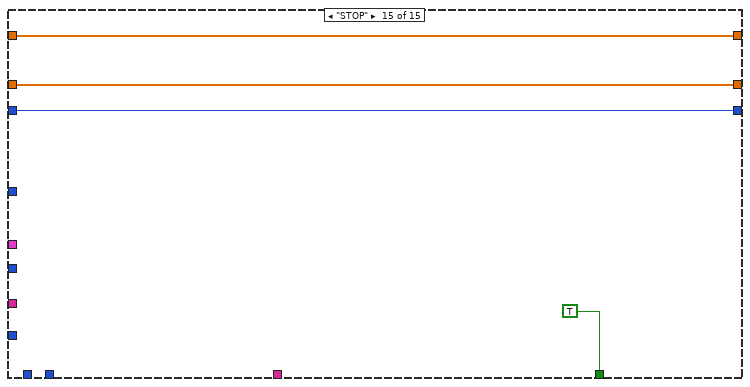
[diagram p20: hidden frame]
diagram:
  w3 = cluster{"String":string, "variant":variant} {"String"="Controllo condizioni iniziali", "variant"=variant} ("element")
  n1 = global write "Global prova in corso.vi" "MISURA RES IN CORSO"(TRUE ("prova in corso?")) -> ()
  n2 = Obtain Queue(name (unnamed)="Misura resistenze", element data type=w3) -> (queue out=w16:refnum<queue>, error out=w17:errorcluster)  [unwired: 3 in, 1 out]
  n3 = Flush Queue(queue=w16, error in (no error)=w17) -> (queue out=w20:refnum<queue>, error out=w15:errorcluster)  [unwired: 1 out]
  n4 = Enqueue Element At Opposite End(queue=w20, element=w3, error in (no error)=w15) -> (queue out=w21:refnum<queue>, error out=w14:errorcluster)  [unwired: 1 in, 1 out]
  n5 = Initialize Array(0.0, "N°rami") -> (w4:dbl[])
  n6 = while {
    tunnel: w21 -> [w48]
    shift-right: [w42] -> _
    shift-left: 0 -> [w38]
    tunnel: w14 -> [w36]
    shift-right: [w33] -> w10
    shift-left: w4 -> [w35]
    shift-right: [w32] -> w13
    shift-left: w4 -> [w34]
    tunnel: "N°rami" -> [w31]
    tunnel: "String" -> [w30]
    tunnel: "Scala di misura" -> [w29]
    tunnel: 0.5 ("Time Target (s)") -> [w26]
    tunnel: "Scala per ramo" -> [w25]
    tunnel: "Status" -> [w22]
    i -> [w28]
    stop <- w44 stop-if-true
    w27 = u32 200 ("millisecond multiple")
    n7 = Dequeue Element(queue=w48, error in (no error)=w36) -> (queue out=w43:refnum<queue>, element=w47:cluster{"String":string, "variant":variant})  [unwired: 1 in, 2 out]
    n8 = global read "Global_All_Data.vi" "All Data"() -> (w24:T5)
    n9 = Increment(x=w38) -> (x+1=w39:i32)
    n10 = Unbundle By Name(w24) -> ("MISURE ALL"=w23:T7)
    n11 = Unbundle By Name(w47) -> ("String"=w46:string, "variant"=w45:variant)
    "Message" <- w46
    n12 = Number To Decimal String(number=w39) -> (decimal integer string=w37:string)  [unwired: 1 in]
    n13 = Wait Until Next ms Multiple(millisecond multiple=w27) -> ()  [unwired: 1 out]
    n14 = case shown="\"Misura!\"" w46 {
      tunnel: w45 -> [_ _ _ _ _ _ _ _ _ w227 _ _ _ _ _]
      tunnel: [_ _ _ _ _ _ _ _ _ _ _ _ _ TRUE TRUE] -> w44
      tunnel: w43 -> [_ w52 w91 w122 w127 w139 w154 w168 _ w225 w233 w247 w258 _ _]
      tunnel: w38 -> [w51 w67 w107 w119 w135 w145 w152 w164 w199 w216 w237 w255 w261 w266 w271]
      tunnel: [w51 w67 w107 w119 w135 w145 w152 w164 w199 w216 w236 w255 w261 w266 w271] -> w42
      tunnel: [_ _ _ "Apertura teleruttore wattmetro" ("string") _ _ "Chiusura teleruttore resistomat" ("string") w161 w203 w222 _ _ _ "Fine" ("string") _] -> w40
      tunnel: w37 -> [_ _ _ _ _ _ _ _ w205 w223 _ _ _ _ _]
      tunnel: w35 -> [w49 w66 w105 w116 w134 w144 w149 w159 w201 w221 w230 w254 w260 w263 w268]
      tunnel: w34 -> [w50 w65 w106 w117 w133 w143 w150 w160 w202 w218 w231 w253 w259 w264 w269]
      tunnel: [w49 w66 w105 w116 w134 w144 w149 w159 w201 w219 w230 w254 w260 w263 w268] -> w33
      tunnel: [w50 w65 w106 w117 w133 w143 w150 w160 w202 w217 w231 w253 w259 w264 w269] -> w32
      tunnel: w31 -> [_ _ _ _ _ _ _ _ _ _ w232 _ _ _ _]
      tunnel: w29 -> [_ _ _ _ _ _ _ _ _ _ _ _ _ _ _]
      tunnel: w28 -> [_ _ w100 _ _ _ _ _ _ _ _ _ _ _ _]
      tunnel: w27 -> [_ _ w101 _ _ _ _ _ _ _ _ _ _ _ _]
      tunnel: w26 -> [_ _ _ _ w132 _ _ _ _ _ _ _ _ _ _]
      tunnel: w25 -> [_ _ _ _ _ _ _ _ w200 _ _ _ _ _ _]
      tunnel: w23 -> [_ w64 w72 w112 w124 w137 w147 w157 _ w211 _ w238 _ _ _]
      frame "False", Default {
      }
      frame "Controllo condizioni iniziali" {
        n15 = Unbundle By Name(w64) -> ("INTERFACCIA.DI (logici).Potenza DC abilitata"=w60:bool, "INTERFACCIA.DI (logici).Ramo 1 resistomat"=w63:bool, "INTERFACCIA.DI (logici).Ramo 2 resistomat"=w62:bool, "INTERFACCIA.DI (logici).Ramo 3 resistomat"=w61:bool)
        n16 = Not(x=w60) -> (.not. x?=w58:bool)
        n17 = Compound Arithmetic op=OR(w63, w62, w61) -> (w59:bool)
        n18 = Not(x=w59) -> (.not. x?=w57:bool)
        n19 = And(x=w57, y=w58) -> (x .and. y?=w56:bool)
        n20 = case shown="True" w59 {
          frame False {
          }
          frame True {
            n21 = call "Set DO.vi"("Cluster SET DO"=T1 [{"DO"=enum."*Abil teler ramo 1 Resist", "Value"=FALSE}, {"DO"=enum."*Abil teler ramo 2 Resist", "Value"=FALSE}, {"DO"=enum."*Abil teler ramo 3 Resist", "Value"=FALSE}]) -> ()  [unwired: 10 in, 1 out]
          }
        }
        n22 = case shown="True" w60 {
          frame False {
          }
          frame True {
            n23 = call "Set DO.vi"("Cluster SET DO"=T1 [{"DO"=enum."OFF: ALL DO", "Value"=FALSE}]) -> ()  [unwired: 10 in, 1 out]
          }
        }
        n24 = Select(t=cluster{"\nStato":string, variant} {"\nStato"="Initialize", variant}, s=w56, f=cluster{"\nStato":string, variant} {"\nStato"="Controllo condizioni iniziali", variant}) -> (s? t:f=w53:cluster{"\nStato":string, variant})
        n25 = Enqueue Element At Opposite End(queue=w52, element=w53) -> ()  [unwired: 2 in, 3 out]
      }
      frame "Initialize" {
        w96 = 10.0  # t max iniz (s)
        w89 = 15.0 ("y")
        n26 = Unbundle By Name(w72) -> ("INTERFACCIA.DI (logici).Teleruttore WT abilitato"=w71:bool)
        n27 = Multiply(x=w101, y=w100) -> (x*y=w99:u32)
        n28 = Unbundle By Name(w72) -> ("INTERFACCIA.DI (logici).Potenza DC abilitata"=w75:bool, "INTERFACCIA.DI (logici).Teleruttore WT abilitato"=w74:bool)
        n29 = case shown="False" w71 {
          frame False {
            # "PER CONTROLLO SU TENSIONI"
            n30 = call "Set DO.vi"("Cluster SET DO"=T1 [{"DO"=enum."*Abilit teler ramo WT", "Value"=TRUE}]) -> ()  [unwired: 10 in, 1 out]
          }
          frame True {
          }
        }
        n31 = global read "Global_scelta_linea.vi" "Linea selezionata"() -> (w73:i16)
        n32 = Unbundle By Name(w72) -> ("INTERFACCIA.AI.RPM"=w81:T14[], "MISURE WT.URMS 1"=w78:dbl, "MISURE WT.URMS 2"=w77:dbl, "MISURE WT.URMS 3"=w76:dbl)
        n33 = Divide(x=w99, y=u32 1000) -> (x/y=w97:dbl)
        n34 = Index Array(array=w81, index=w73) -> (element=w80:T14)
        n35 = Unbundle By Name(w80) -> ("Misura"=w79:dbl)
        n36 = Greater?(x=w97, y=w96) -> (0:w95:bool)
        n37 = Not(x=w75) -> (.not. x?=w90:bool)
        n38 = Less?(x=w79, y=w89) -> ()  [unwired: 1 out]
        n39 = Less?(x=w78, y=w89) -> (x < y?=w104:bool)
        n40 = Less?(x=w77, y=w89) -> (x < y?=w88:bool)
        n41 = Less?(x=w76, y=w89) -> (x < y?=w87:bool)
        n42 = Compound Arithmetic op=AND(TRUE ("value"), w104, w90, w88, w87, w74) -> (w85:bool)
        n43 = Not(x=w85) -> (.not. x?=w84:bool)
        n44 = call "Elapsed Time2"("Time Target (s)"=3.0, "Reset"=w84, "Auto Reset"=FALSE) -> ("Time has Elapsed"=w82:bool)  [unwired: 9 in, 7 out]
        n45 = Select(t=cluster{"\nStato":string, variant} {"\nStato"="Apri telerutt wt", variant}, s=w82, f=cluster{"\nStato":string, variant} {"\nStato"="Initialize", variant}) -> (s? t:f=w94:cluster{"\nStato":string, variant})
        n46 = Select(t=cluster{"\nStato":string, variant} {"\nStato"="Fine prova", variant}, s=w95, f=w94) -> (s? t:f=w93:cluster{"\nStato":string, variant})
        n47 = Enqueue Element At Opposite End(queue=w91, element=w93) -> ()  [unwired: 2 in, 3 out]
      }
      frame "Apri telerutt wt" {
        # "controlla che il teleruttore del wt sia aperto\ne che tutti i teleruttori di potenza siano aperti"
        n48 = Unbundle By Name(w112) -> ("INTERFACCIA.DI (logici).Teleruttore WT abilitato"=w111:bool, "INTERFACCIA.DI (logici).Potenza trifase abilitata"=w110:bool, "INTERFACCIA.DI (logici).Potenza monofase abilitata"=w109:bool)
        n49 = Compound Arithmetic op=OR(w111, w110, w109) -> (w114:bool)
        n50 = Select(t=cluster{"\nStato":string, variant} {"\nStato"="Apri telerutt wt", variant}, s=w114, f=cluster{"\nStato":string, variant} {"\nStato"="Corto fasi ON", variant}) -> (s? t:f=w120:cluster{"\nStato":string, variant})
        n51 = call "Set DO.vi"("Cluster SET DO"=T1 [{"DO"=enum."*Disabilita teleruttori potenza", "Value"=FALSE}]) -> ()  [unwired: 10 in, 1 out]
        n52 = Enqueue Element At Opposite End(queue=w122, element=w120) -> ()  [unwired: 2 in, 3 out]
      }
      frame "Corto fasi ON" {
        n53 = Unbundle By Name(w124) -> ("INTERFACCIA.DI (logici).Teleruttore corto fasi"=w123:bool)
        n54 = Not(x=w123) -> (.not. x?=w131:bool)
        n55 = call "Elapsed Time"("Time Target (s)"=w132, "Reset"=w131) -> ("Time has Elapsed"=w125:bool)  [unwired: 10 in, 7 out]
        n56 = call "Set DO.vi"("Cluster SET DO"=T1 [{"DO"=enum."*Abil cortocirc avvolgim", "Value"=TRUE}]) -> ()  [unwired: 10 in, 1 out]
        n57 = Select(t=cluster{"\nStato":string, variant} {"\nStato"="Corto fasi OFF", variant}, s=w125, f=cluster{"\nStato":string, variant} {"\nStato"="Corto fasi ON", variant}) -> (s? t:f=w128:cluster{"\nStato":string, variant})
        n58 = Enqueue Element At Opposite End(queue=w127, element=w128) -> ()  [unwired: 2 in, 3 out]
      }
      frame "Corto fasi OFF" {
        n59 = Unbundle By Name(w137) -> ("INTERFACCIA.DI (logici).Teleruttore corto fasi"=w136:bool)
        n60 = call "Set DO.vi"("Cluster SET DO"=T1 [{"DO"=enum."*Abil cortocirc avvolgim", "Value"=FALSE}]) -> ()  [unwired: 10 in, 1 out]
        n61 = Select(t=cluster{"\nStato":string, variant} {"\nStato"="Corto fasi OFF", variant}, s=w136, f=cluster{"\nStato":string, variant} {"\nStato"="Chiudi tel principale resistomat", variant}) -> (s? t:f=w140:cluster{"\nStato":string, variant})
        n62 = Enqueue Element At Opposite End(queue=w139, element=w140) -> ()  [unwired: 2 in, 3 out]
      }
      frame "Chiudi tel principale resistomat" {
        # "controlla chiusura tel principale resistomat"
        # "Chiudi telertuttore principale resistomat"
        n63 = Unbundle By Name(w147) -> ("INTERFACCIA.DI (logici).Teleruttore Resistomat abilitato"=w146:bool)
        n64 = call "Set DO.vi"("Cluster SET DO"=T1 [{"DO"=enum."*Abil teler ramo princ Resit", "Value"=TRUE}]) -> ()  [unwired: 10 in, 1 out]
        n65 = Select(t=cluster{"\nStato":string, variant} {"\nStato"="Chiudi ramo", variant}, s=w146, f=cluster{"\nStato":string, variant} {"\nStato"="Chiudi tel principale resistomat", variant}) -> (s? t:f=w155:cluster{"\nStato":string, variant})
        n66 = Enqueue Element At Opposite End(queue=w154, element=w155) -> ()  [unwired: 2 in, 3 out]
      }
      frame "Chiudi ramo" {
        n67 = Increment(x=w164) -> (x+1=w163:i32)
        n68 = case shown="0, Default" w164 {
          tunnel: [w177 w183 w191] -> w158
          tunnel: w157 -> [w172 w181 w186]
          frame 0, Default {
            # "controlla chiusura tel ramo 1"
            n69 = Unbundle By Name(w172) -> ("INTERFACCIA.DI (logici).Ramo 1 resistomat"=w175:bool, "INTERFACCIA.DI (logici).Ramo 2 resistomat"=w171:bool, "INTERFACCIA.DI (logici).Ramo 3 resistomat"=w170:bool)
            n70 = Not(x=w171) -> (.not. x?=w174:bool)
            n71 = Not(x=w170) -> (.not. x?=w173:bool)
            n72 = call "Set DO.vi"("Cluster SET DO"=T1 [{"DO"=enum."*Abil teler ramo 1 Resist", "Value"=TRUE}, {"DO"=enum."*Abil teler ramo 2 Resist", "Value"=FALSE}, {"DO"=enum."*Abil teler ramo 3 Resist", "Value"=FALSE}]) -> ()  [unwired: 10 in, 1 out]
            n73 = Compound Arithmetic op=AND(w175, w174, w173) -> (w177:bool)
          }
          frame 1 {
            n74 = Unbundle By Name(w181) -> ("INTERFACCIA.DI (logici).Ramo 1 resistomat"=w180:bool, "INTERFACCIA.DI (logici).Ramo 2 resistomat"=w179:bool, "INTERFACCIA.DI (logici).Ramo 3 resistomat"=w178:bool)
            n75 = call "Set DO.vi"("Cluster SET DO"=T1 [{"DO"=enum."*Abil teler ramo 1 Resist", "Value"=FALSE}, {"DO"=enum."*Abil teler ramo 2 Resist", "Value"=TRUE}, {"DO"=enum."*Abil teler ramo 3 Resist", "Value"=FALSE}]) -> ()  [unwired: 10 in, 1 out]
            n76 = Not(x=w180) -> (.not. x?=w184:bool)
            n77 = Not(x=w178) -> (.not. x?=w185:bool)
            n78 = Compound Arithmetic op=AND(w184, w179, w185) -> (w183:bool)
          }
          frame 2 {
            n79 = Unbundle By Name(w186) -> ("INTERFACCIA.DI (logici).Ramo 1 resistomat"=w187:bool, "INTERFACCIA.DI (logici).Ramo 2 resistomat"=w188:bool, "INTERFACCIA.DI (logici).Ramo 3 resistomat"=w189:bool)
            n80 = call "Set DO.vi"("Cluster SET DO"=T1 [{"DO"=enum."*Abil teler ramo 1 Resist", "Value"=FALSE}, {"DO"=enum."*Abil teler ramo 2 Resist", "Value"=FALSE}, {"DO"=enum."*Abil teler ramo 3 Resist", "Value"=TRUE}]) -> ()  [unwired: 10 in, 1 out]
            n81 = Not(x=w187) -> (.not. x?=w193:bool)
            n82 = Not(x=w188) -> (.not. x?=w192:bool)
            n83 = Compound Arithmetic op=AND(w193, w192, w189) -> (w191:bool)
          }
        }
        n84 = Number To Decimal String(number=w163) -> (decimal integer string=w162:string)  [unwired: 1 in]
        n85 = Concatenate Strings("Chiusura ramo n°" ("string"), w162) -> (w161:string)
        n86 = Select(t=cluster{"\nStato":string, variant} {"\nStato"="Misura!", variant}, s=w158, f=cluster{"\nStato":string, variant} {"\nStato"="Chiudi ramo", variant}) -> (s? t:f=w169:cluster{"\nStato":string, variant})
        n87 = Enqueue Element At Opposite End(queue=w168, element=w169) -> ()  [unwired: 2 in, 3 out]
      }
      frame "Misura!" {
        n88 = Index Array(array=w200, index=w199) -> (element=w196:i32)
        n89 = Concatenate Strings("Misura n°" ("string"), w205, " in corso" ("string")) -> (w203:string)
        n90 = Bundle By Name(cluster=T4 {"Array of elements"=[], "Single element"={"String"="START RES", "variant"=variant}, "enque at\nopposite end (F)"=FALSE, "no replications (F)"=FALSE} ("Enqueue cluster"), "Single element.variant"=w196) -> (w195:T4)
        n91 = call <userlib>:"SMQ_MANAGER.vi"("Function"=enum16{"INITIALIZE", "ENQUEUE", "STOP ALL"}."ENQUEUE", "Queue name"="RES_Q", "Enqueue cluster"=w195) -> ()  [unwired: 8 in, 1 out]
      }
      frame "Acquisisci misura res" {
        w208 = 0  # index Tamb [°C]
        # "Tamb"
        # "Attendi misura del resistomat.\n\nLa lettura viene inviata in questo case\ndal RES.vi una volta che la lettura è pronta"
        n92 = Unbundle By Name(w211) -> ("INTERFACCIA.AI.Temperature"=w210:T14[])
        n93 = Variant To Data(type=0.0, Variant=w227) -> (data=w220:dbl)  [unwired: 1 in, 1 out]
        n94 = Concatenate Strings("Acquisizione misura n°" ("string"), w223) -> (w222:string)
        n95 = Index Array(array=w210, index=w208) -> (element=w209:T14)
        n96 = Unbundle By Name(w209) -> ("Misura"=w207:dbl)
        n97 = Replace Array Subset(array=w221, new element=w220, index=w216) -> (w219:dbl[])
        n98 = Replace Array Subset(array=w218, new element=w207, index=w216) -> (w217:dbl[])
        n99 = global read "Stop lettura res.vi" "STOP LETTURA RES"() -> (w215:bool)
        n100 = Select(t=cluster{"String":string, "variant":variant} {"String"="Disabilita prova", "variant"=variant} ("element"), s=w215, f=cluster{"String":string, "variant":variant} {"String"="Incrementa ramo", "variant"=variant} ("element")) -> (s? t:f=w214:cluster{"String":string, "variant":variant})
        n101 = Enqueue Element(queue=w225, element=w214) -> ()  [unwired: 2 in, 3 out]
      }
      frame "Incrementa ramo" {
        n102 = Increment(x=w237) -> (x+1=w236:i32)
        n103 = Greater Or Equal?(x=w236, y=w232) -> (x >= y?=w235:bool)
        n104 = Select(t=cluster{"String":string, "variant":variant} {"String"="Disabilita prova", "variant"=variant} ("element"), s=w235, f=cluster{"String":string, "variant":variant} {"String"="Chiudi ramo", "variant"=variant} ("element")) -> (s? t:f=w234:cluster{"String":string, "variant":variant})
        n105 = Enqueue Element(queue=w233, element=w234) -> ()  [unwired: 2 in, 3 out]
      }
      frame "Disabilita prova" {
        n106 = Unbundle By Name(w238) -> ("INTERFACCIA.DI (logici).Teleruttore Resistomat abilitato"=w242:bool, "INTERFACCIA.DI (logici).Ramo 1 resistomat"=w241:bool, "INTERFACCIA.DI (logici).Ramo 2 resistomat"=w240:bool, "INTERFACCIA.DI (logici).Ramo 3 resistomat"=w239:bool)
        n107 = Not(x=w242) -> (.not. x?=w249:bool)
        n108 = Not(x=w241) -> (.not. x?=w250:bool)
        n109 = Not(x=w240) -> (.not. x?=w252:bool)
        n110 = Not(x=w239) -> (.not. x?=w251:bool)
        n111 = Compound Arithmetic op=AND(w249, w250, w252, w251) -> (w246:bool)
        n112 = Select(t=cluster{"String":string, "variant":variant} {"String"="Inserisci WT", "variant"=variant} ("element"), s=w246, f=cluster{"String":string, "variant":variant} {"String"="Disabilita prova", "variant"=variant} ("element")) -> (s? t:f=w248:cluster{"String":string, "variant":variant})
        n113 = call "Set DO.vi"("Cluster SET DO"=T1 [{"DO"=enum."*Abil teler ramo 1 Resist", "Value"=FALSE}, {"DO"=enum."*Abil teler ramo 2 Resist", "Value"=FALSE}, {"DO"=enum."*Abil teler ramo 3 Resist", "Value"=FALSE}, {"DO"=enum."*Abil teler ramo princ Resit", "Value"=FALSE}]) -> ()  [unwired: 10 in, 1 out]
        n114 = Enqueue Element(queue=w247, element=w248) -> ()  [unwired: 2 in, 3 out]
      }
      frame "Inserisci WT" {
        n115 = call "Set DO.vi"("Cluster SET DO"=T1 [{"DO"=enum."*Abilit teler ramo WT", "Value"=FALSE}]) -> ()  [unwired: 10 in, 1 out]
        n116 = Enqueue Element(queue=w258, element=cluster{"String":string, "variant":variant} {"String"="Fine prova", "variant"=variant}) -> ()  [unwired: 2 in, 3 out]
      }
      frame "Fine prova" {
        n117 = global write "Global prova in corso.vi" "MISURA RES IN CORSO"(FALSE ("prova in corso?")) -> ()
      }
      frame "STOP" {
      }
    }
    n118 = Concatenate Strings(w30, w40) -> (w41:string)
    n119 = property class="Str"(reference=w22, "Value"=w41) -> ()  [unwired: 1 in, 2 out]
  }
  "Valori res (ohm)" <- w10
  "temperature amb" <- w13
  n120 = call-poly <vilib>:"Mean.vi"("X"=w10) -> ("mean"=→"Rmedia (ohm)":dbl)  [unwired: 1 out]
